vi "Add Monitor Recorders.vi"(6 "Reset":bool, 8 "error in (no error)":errorcluster, 10 "Module type":T1, 11 "Monitor-Pulse in":refnum<class "Application Controller.lvclass">) -> (0 "error out":errorcluster, 2 "Actot names out":string[](array[string]), 3 "Monitor-Pulse out":refnum<class "Application Controller.lvclass">)   [LabVIEW 2019, in "Application Controller.lvclass"]
uses:
  Application Controller.lvclass
  Module Types.ctl
  Instrument Actor/Instrument Actor.lvclass
  C:/GitHub/LabActor/Worker/Worker.lvclass
  Recorders/Micron Optics/Micron Optics Recorder.lvclass
  C:/GitHub/LabActor/Recorders/Spectrometer/Spectrometer.lvclass
  NHMFL_Core/Libraries/Instruments/Micron Optics/Micron Hyperion Driver/Micron Hyperion Driver.lvclass
  C:/GitHub/NHMFL_Core/Libraries/Instruments/Spectrometer Driver/Spectrometer Driver.lvclass
  Spectrum Recorder too/Spectrum Recorder too.lvclass
  C:/GitHub/LabActor/Instrument Actor/Instrument Actor.lvclass
  NHMFL_Core/Libraries/Red Pitaya/RP Core/Red Pitaya Transceiver Driver/Red Pitaya Transceiver Driver.lvclass
  C:/GitHub/NHMFL_Core/Libraries/Instruments/Instrument Driver/Instrument Driver.lvclass
  Instrument Actor/Instrument Actor.lvclass/Instrument Actor.ctl
  Post-Processors/Elastic Moduli/Format Resonances.lvclass
  Application Controller.lvclass/Application Controller.ctl
  Instrument Actor/Write Instrument driver.vi
  Read Monitor ref.vi
  Write Monitor ref.vi
  Worker/Worker.lvclass
  C:/GitHub/LabActor/Template Module/Template Module.lvclass
  Recorders/Spectrometer/Write Spectrometer Driver.lvclass.vi
  NHMFL_Core/Libraries/Queued Listbox/Queued Listbox.xctl
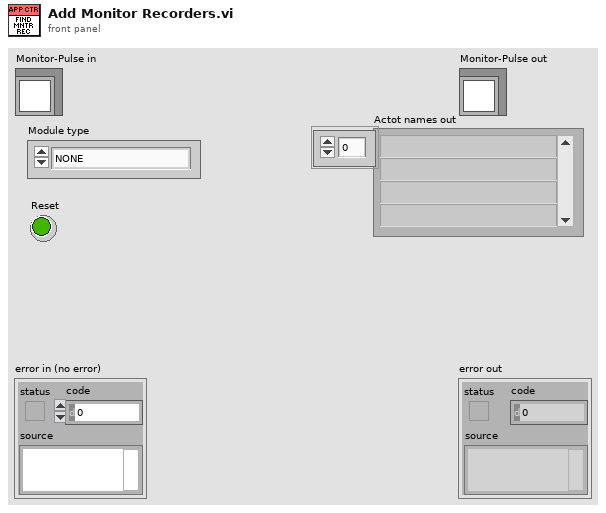
[diagram p1: front panel]
types:
  T1 = typedef "Module Types.ctl" = enum16{"NONE", "NI-DAQmx", "NI-Scope", "Red Pitaya Digitizer", "GaGe", "VISA Device", "Red Pitaya Lockin", "Monitor Controller", "Pulse Controller", "Integrate Pulse", "Lockin Processor", "File converter", "NHMFL Synthesizer", "Micron Hyperion", "Spectrum Recorder", "Resonance Detector", "TCP Communications", "Format Resonances", "Ruby Spectra", "PID Controller", "Quantum Design", "VI Server"}
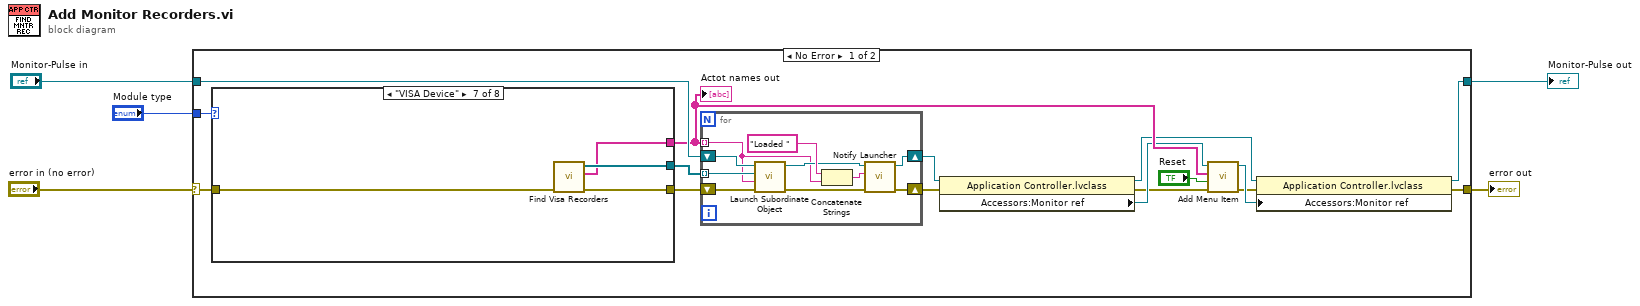
[diagram p0: block diagram]
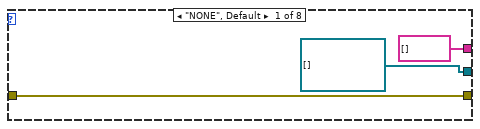
[diagram p2: hidden frame]
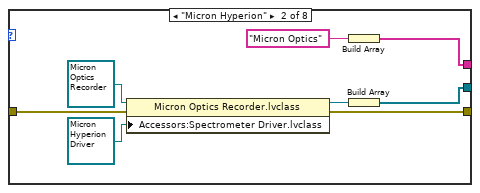
[diagram p3: hidden frame]
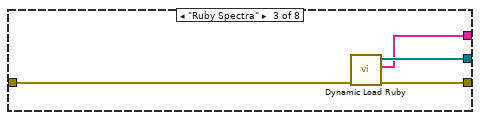
[diagram p4: hidden frame]
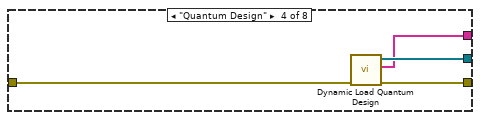
[diagram p5: hidden frame]
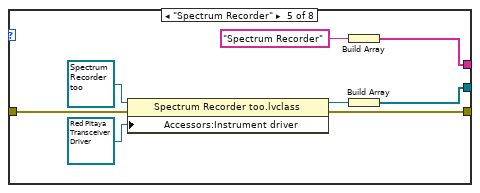
[diagram p6: hidden frame]
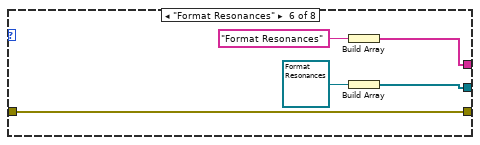
[diagram p7: hidden frame]
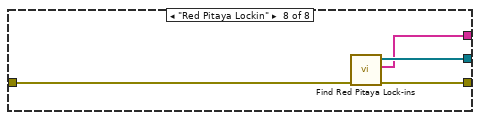
[diagram p8: hidden frame]
diagram:
  n1 = case shown="No Error" "error in (no error)" {
    selector: "error in (no error)" -> [w21 w73]
    tunnel: [w6 w73] -> w4
    tunnel: [w12 w72] -> w2
    tunnel: "Monitor-Pulse in" -> [w20 w72]
    tunnel: "Module type" -> [w17 _]
    frame No Error {
      n2 = case shown="\"VISA Device\"" w17 {
        tunnel: w21 -> [w22 w31 w36 w40 w47 w52 w57 w60]
        tunnel: [refnum<class "Instrument Actor.lvclass">[] [] ("Recorders List") w32 w34 w38 w48 w53 w56 w59] -> w19
        tunnel: [string[] [] ("Names") w25 w33 w37 w41 w49 w55 w58] -> w15
        tunnel: [w22 w30 w35 w39 w46 w52 w54 w61] -> w18
        frame "NONE", Default {
        }
        frame "Micron Hyperion" {
          n3 = property class="Micron Optics Recorder.lvclass"(reference=refnum<class "Micron Optics Recorder.lvclass"> refnum ("Micron Optics Recorder.lvclass"), error in=w31, "Accessors:Spectrometer Driver.lvclass"=refnum<class "Micron Hyperion Driver.lvclass"> refnum ("Micron Hyperion Driver.lvclass")) -> (reference out=w28:refnum<class "Micron Optics Recorder.lvclass">, error out=w30:errorcluster)
          n4 = Build Array("Micron Optics") -> (w25:string[])
          n5 = Build Array(w28) -> (w32:refnum<class "Micron Optics Recorder.lvclass">[])
        }
        frame "Ruby Spectra" {
          n6 = call "Dynamic Load Ruby.vi"("Error In"=w36) -> ("Error Out"=w35:errorcluster, "Device names"=w33:string[], "Digitizers out"=w34:refnum<class "Instrument Actor.lvclass">[])  [unwired: 8 in]
        }
        frame "Quantum Design" {
          n7 = call "Dynamic Load Quantum Design.vi"("Error In"=w40) -> ("Error Out"=w39:errorcluster, "Device names"=w37:string[], "Digitizers out"=w38:refnum<class "Instrument Actor.lvclass">[])  [unwired: 8 in]
        }
        frame "Spectrum Recorder" {
          n8 = property class="Spectrum Recorder too.lvclass"(reference=refnum<class "Spectrum Recorder too.lvclass"> refnum ("Spectrum Recorder too.lvclass"), error in=w47, "Accessors:Instrument driver"=refnum<class "Red Pitaya Transceiver Driver.lvclass"> refnum ("Red Pitaya Transceiver Driver.lvclass")) -> (reference out=w44:refnum<class "Spectrum Recorder too.lvclass">, error out=w46:errorcluster)
          n9 = Build Array("Spectrum Recorder") -> (w41:string[])
          n10 = Build Array(w44) -> (w48:refnum<class "Spectrum Recorder too.lvclass">[])
        }
        frame "Format Resonances" {
          n11 = Build Array("Format Resonances") -> (w49:string[])
          n12 = Build Array(refnum<class "Format Resonances.lvclass"> refnum ("Elastic Moduli.lvclass")) -> (w53:refnum<class "Format Resonances.lvclass">[])
        }
        frame "VISA Device" {
          n13 = call "Find Visa Recorders.vi"("Error In"=w57) -> ("Error Out"=w54:errorcluster, "Names"=w55:string[], "Recorders List"=w56:refnum<class "Instrument Actor.lvclass">[])  [unwired: 8 in]
        }
        frame "Red Pitaya Lockin" {
          n14 = call "Find Red Pitaya Lock-ins.vi"("Error In"=w60) -> ("Error Out"=w61:errorcluster, "Names"=w58:string[], "Instruments out"=w59:refnum<class "Instrument Actor.lvclass">[])  [unwired: 7 in, 1 out]
        }
      }
      "Actot names out" <- w15
      n15 = for {
        shift-right: [w65] -> w16
        shift-left: w20 -> [w71]
        shift-right: [w63] -> w9
        shift-left: w18 -> [w70]
        tunnel: w19 -> [w69] mode=indexing
        tunnel: w15 -> [w62] mode=indexing
        n16 = call-dynamic "Launch Subordinate Object.vi"("error in (no error)"=w70, "Name"=w62, "Subordinate Object"=w69, "Measure Object in"=w71) -> ("error out"=w64:errorcluster, "Measure Object out"=w66:refnum<class "Application Controller.lvclass">)  [unwired: 5 in, 1 out]
        n17 = Concatenate Strings("Loaded " ("string"), w62) -> (w67:string)
        n18 = call-dynamic "Notify Launcher.vi"("error in (no error)"=w64, "Notification"=w67, "Application Controller in"=w66) -> ("error out"=w63:errorcluster, "Application Controller out"=w65:refnum<class "Application Controller.lvclass">)  [unwired: 7 in]
      }
      n19 = property class="Application Controller.lvclass"(reference=w16, error in=w9) -> (reference out=w13:refnum<class "Application Controller.lvclass">, error out=w8:errorcluster, "Accessors:Monitor ref"=w11:refnum<vi>)
      n20 = call "Add Menu Item.vi"("error in (no error)"=w8, "Reset"="Reset", "Item Names"=w15, "Queed Listbox ref"=w11) -> ("error out"=w7:errorcluster, "Queed Listbox ref out"=w10:refnum<vi>)  [unwired: 5 in, 1 out]
      n21 = property class="Application Controller.lvclass"(reference=w13, error in=w7, "Accessors:Monitor ref"=w10) -> (reference out=w12:refnum<class "Application Controller.lvclass">, error out=w6:errorcluster)
    }
    frame Error {
    }
  }
  "error out" <- w4
  "Monitor-Pulse out" <- w2
